vi "Get Root Directory Ref(冲突时的文件备份2013-03-27 14-07-54).vi"(8 "error in (no error)":errorcluster caption="错误输入（无错误）", 11 "DriveInfo 输入":refnum<class "DriveInfo.lvclass"> caption="DNL_LabVIEW Object in") -> (0 "error out":errorcluster caption="错误输出", 3 "DriveInfo 输出":refnum<class "DriveInfo.lvclass"> caption="DNL_LabVIEW Object out")   [LabVIEW 2012, in "DriveInfo.lvclass"]
uses:
  DriveInfo.lvclass
  DriveInfo.lvclass/DriveInfo.ctl
panel:
  out "RootDirectory":refnum<k24>
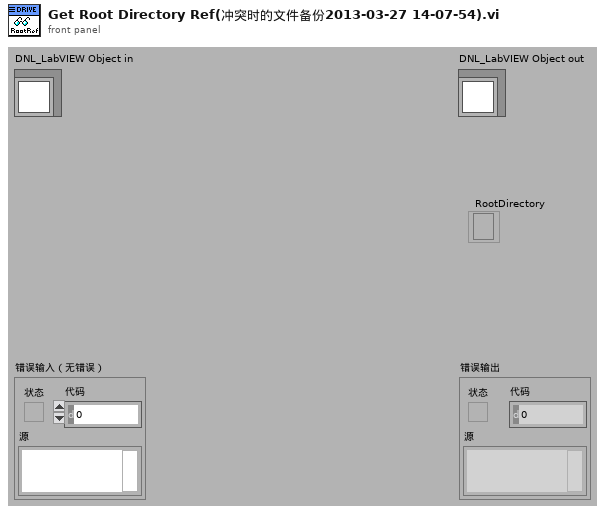
[diagram p1: front panel]
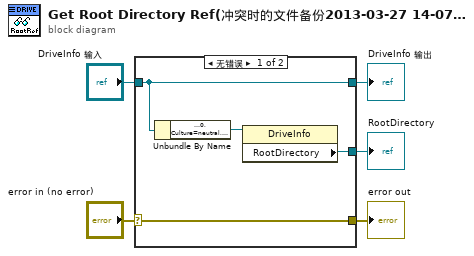
[diagram p0: block diagram]
diagram:
  n1 = case shown="无错误" "error in (no error)" {
    selector: "error in (no error)" -> [w9 w11]
    tunnel: [w9 w11] -> w4
    tunnel: [w8 w10] -> w2
    tunnel: "DriveInfo 输入" -> [w8 w10]
    tunnel: [w6 _] -> w1
    frame No Error {
      n2 = Unbundle By Name(w8) -> ("DriveInfo"=w7:refnum<k24>)
      n3 = property class="DriveInfo"(reference=w7) -> ("RootDirectory"=w6:refnum<k24>)  [unwired: 1 in, 2 out]
    }
    frame Error {
    }
  }
  "error out" <- w4
  "DriveInfo 输出" <- w2
  "RootDirectory" <- w1
